vi "macro_SwerveDriveOdomNew4.vi"   [LabVIEW 2019, in "Trajectory_Library.lvlib"]
uses:
  Trajectory_Library.lvlib
types:
  T1 = typedef "Trajectory_Library.lvlib/ROTATION2D.ctl" = cluster{"VALUE":dbl, "COS":dbl, "SIN":dbl}
  T2 = typedef "WPILib_Math.lvlib/SWERVE_DRIVE_MODULE_POSITION.ctl" = cluster{"Distance":dbl, "Angle":T3, "P":bool}
  T3 = typedef "WPILib_Math.lvlib/ROTATION2D.ctl" = cluster{"VALUE":dbl, "COS":dbl, "SIN":dbl}
  T4 = typedef "Trajectory_Library.lvlib/POSE2D.ctl" = cluster{"TRANSLATION":T5, "ROTATION":T1}
  T5 = typedef "Trajectory_Library.lvlib/TRANSLATION2D.ctl" = cluster{"X":dbl, "Y":dbl}
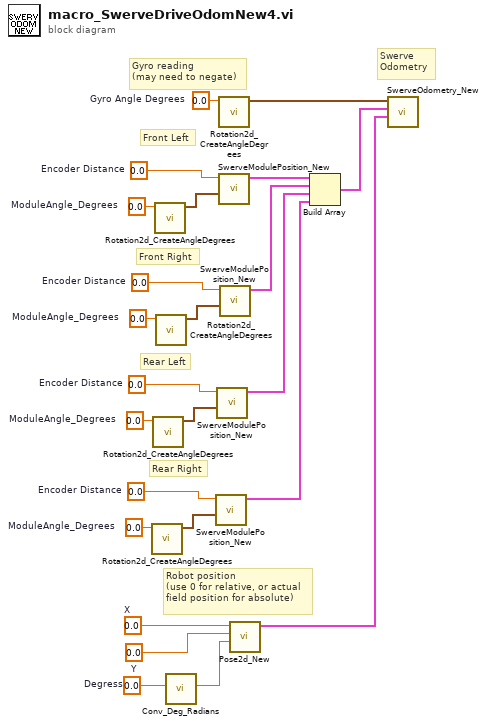
[diagram p0: block diagram]
diagram:
  w2 = 0.0  # Degress
  w3 = 0.0  # X
  w4 = 0.0  # Y
  w11 = 0.0  # ModuleAngle_Degrees
  w13 = 0.0  # Encoder Distance
  w14 = 0.0  # ModuleAngle_Degrees
  w16 = 0.0  # Encoder Distance
  w17 = 0.0  # ModuleAngle_Degrees
  w19 = 0.0  # Encoder Distance
  w21 = 0.0  # Gyro Angle Degrees
  w22 = 0.0  # ModuleAngle_Degrees
  w24 = 0.0  # Encoder Distance
  # "Swerve\nOdometry"
  # "Robot position\n(use 0 for relative, or actual \nfield position for absolute)"
  # "Rear Right"
  # "Rear Left"
  # "Front Right"
  # "Front Left"
  # "Gyro reading\n(may need to negate)"
  n1 = call "Rotation2d_CreateAngleDegrees.vi"("Angle_Degrees"=w11) -> ("ROTATION"=w12:T1)  [unwired: 10 in]
  n2 = call "Rotation2d_CreateAngleDegrees.vi"("Angle_Degrees"=w14) -> ("ROTATION"=w15:T1)  [unwired: 10 in]
  n3 = call "Rotation2d_CreateAngleDegrees.vi"("Angle_Degrees"=w22) -> ("ROTATION"=w23:T1)  [unwired: 10 in]
  n4 = call "Rotation2d_CreateAngleDegrees.vi"("Angle_Degrees"=w17) -> ("ROTATION"=w18:T1)  [unwired: 10 in]
  n5 = call "Conv_Deg_Radians.vi"("Degress"=w2) -> ("Radians"=w5:dbl)  [unwired: 10 in]
  n6 = call "SwerveModulePosition_New.vi"("ROTATION"=w12, "Distance"=w13) -> ("SWERVE_DRIVE_MODULE_POSITION"=w8:T2)  [unwired: 9 in]
  n7 = call "SwerveModulePosition_New.vi"("ROTATION"=w15, "Distance"=w16) -> ("SWERVE_DRIVE_MODULE_POSITION"=w9:T2)  [unwired: 9 in]
  n8 = call "Rotation2d_CreateAngleDegrees.vi"("Angle_Degrees"=w21) -> ("ROTATION"=w7:T1)  [unwired: 10 in]
  n9 = call "SwerveModulePosition_New.vi"("ROTATION"=w23, "Distance"=w24) -> ("SWERVE_DRIVE_MODULE_POSITION"=w20:T2)  [unwired: 9 in]
  n10 = call "SwerveModulePosition_New.vi"("ROTATION"=w18, "Distance"=w19) -> ("SWERVE_DRIVE_MODULE_POSITION"=w10:T2)  [unwired: 9 in]
  n11 = call "Pose2d_New.vi"("Heading"=w5, "Y"=w4, "X"=w3) -> ("out POSe"=w1:T4)  [unwired: 8 in]
  n12 = Build Array(w20, w10, w9, w8) -> (w6:T2[])
  n13 = call "SwerveOdometry_New.vi"("InitialPose"=w1, "Module Positions"=w6, "gyroAngle"=w7) -> ()  [unwired: 8 in, 1 out]
